vi "GetVariables.vi"(8 "error in (no error)":errorcluster, 10 "VariableType":enum16{"String", "StringArray"}(ring), 11 "DicRef":T1) -> (0 "error out":errorcluster, 3 "VariableArray":string[](array[string]))   [LabVIEW 2018]
uses:
  <userlib>/_OpenG.lib/dictionary/dictionary.llb/Dictionary Object RefNum__ogtk.ctl
  <userlib>/_OpenG.lib/dictionary/dictionary.llb/Dictionary Object RefNum - Enum__ogtk.ctl
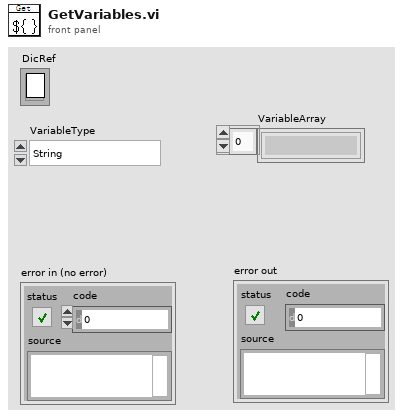
[diagram p1: front panel]
types:
  T1 = typedef "Dictionary Object RefNum__ogtk.ctl" = refnum<k1>
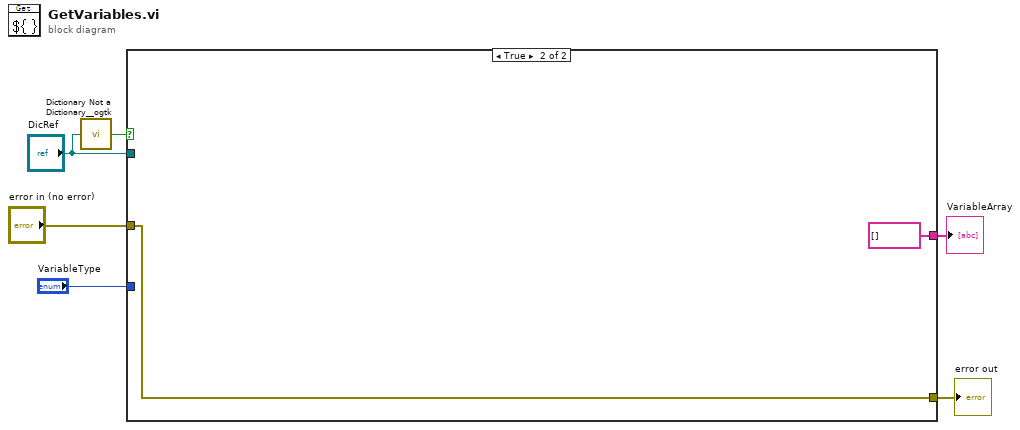
[diagram p0: block diagram]
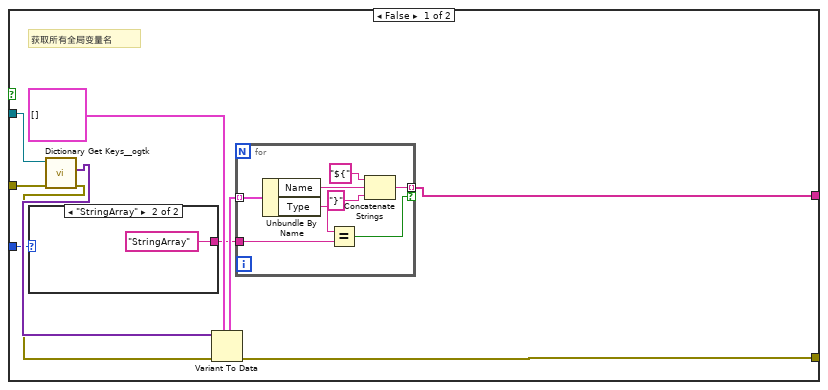
[diagram p2: hidden frame]
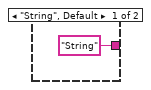
[diagram p3: hidden frame]
diagram:
  n1 = call <userlib>:"Dictionary Not a Dictionary__ogtk.vi"("dictionary"="DicRef") -> ("not a dictionary?"=w4:bool)
  n2 = case shown="True" w4 {
    tunnel: "DicRef" -> [w15 _]
    tunnel: "error in (no error)" -> [w14 w28]
    tunnel: [w10 w28] -> w2
    tunnel: "VariableType" -> [w9 _]
    tunnel: [w7 string[] []] -> w1
    frame False {
      # "获取所有全局变量名"
      n3 = case shown="\"StringArray\"" w9 {
        tunnel: ["String" "StringArray"] -> w8
        frame "String", Default {
        }
        frame "StringArray" {
        }
      }
      n4 = call <userlib>:"Dictionary Get Keys__ogtk.vi"("error in (no error)"=w14, "dictionary"=w15) -> ("error out"=w13:errorcluster, "keys"=w16:variant[])  [unwired: 7 in, 1 out]
      n5 = Variant To Data(error in=w13, type=cluster{"Type":string, "Name":string}[] [] ("VariableArray"), Variant=w16) -> (data=w11:cluster{"Type":string, "Name":string}[], error out=w10:errorcluster)
      n6 = for {
        tunnel: w11 -> [w26] mode=indexing
        tunnel: [w20] -> w7 mode=indexing if=w23
        tunnel: w8 -> [w19]
        n7 = Unbundle By Name(w26) -> ("Name"=w24:string, "Type"=w25:string)
        n8 = Equal?(x=w25, y=w19) -> (x = y?=w23:bool)
        n9 = Concatenate Strings("${" ("string"), w24, "}" ("string")) -> (w20:string)
      }
    }
    frame True {
    }
  }
  "error out" <- w2
  "VariableArray" <- w1
